vi "OSU100_Connect.vi"(8 "error in (no error)":errorcluster, 9 "DeviceName":string) -> (0 "error out":errorcluster, 3 "Reference out":refnum<k24>)   [LabVIEW 2017]
uses:
  C:/Users/Ssantec_Test/Documents/Instrument_DLL_Sample_Labview_20250826_Ver1.5.0_x64/DLL/InstrumentDLL.dll
  DLL/InstrumentDLL.dll
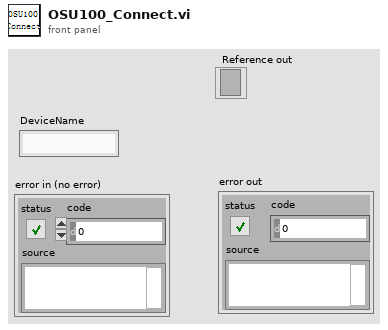
[diagram p1: front panel]
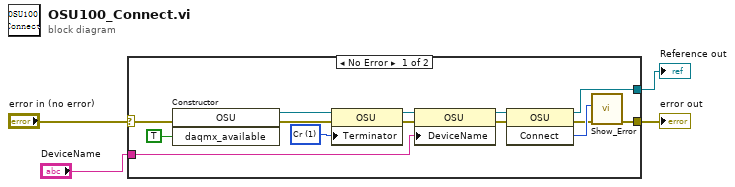
[diagram p0: block diagram]
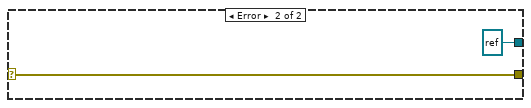
[diagram p2: hidden frame]
diagram:
  n1 = case shown="No Error" "error in (no error)" {
    selector: "error in (no error)" -> [w9 w20]
    tunnel: "DeviceName" -> [w8 _]
    tunnel: [w18 refnum<k24> refnum ("new reference")] -> w3
    tunnel: [w15 w20] -> w1
    frame No Error {
      w12 = 1 items=["CrLf", "Cr", "Lf"] ("Terminator")
      n2 = constructor class="OSU"(error in=w9, "daqmx_available"=TRUE) -> (reference out=w14:refnum<k24>, error out=w13:errorcluster)  [unwired: 2 in, 2 out]
      n3 = property on="属性节点" class="OSU"(reference=w14, error in=w13, "Terminator"=w12) -> (reference out=w11:refnum<k24>, error out=w7:errorcluster)
      n4 = property on="属性节点" class="OSU"(reference=w11, error in=w7, "DeviceName"=w8) -> (reference out=w10:refnum<k24>, error out=w6:errorcluster)
      n5 = invoke on="调用节点" class="OSU" method="Connect"(reference=w10, error in=w6) -> (reference out=w18:refnum<k24>, error out=w16:errorcluster, "Connect"=w17:i32)  [unwired: 1 in]
      n6 = call "Show_Error.vi"("error in (no error)"=w16, "Error"=w17) -> ("error out"=w15:errorcluster)  [unwired: 9 in]
    }
    frame Error {
    }
  }
  "error out" <- w1
  "Reference out" <- w3
